vi "Destroy.vi"(8 "error in (no error)":errorcluster, 11 "StartupSplash in":refnum<class "StartupSplash.lvclass">) -> (0 "error out":errorcluster)   [LabVIEW 2025, in "StartupSplash.lvclass"]
uses:
  StartupSplash.lvclass
  StartupSplash.lvclass/StartupSplash.ctl
  zeromq/Send_string.vi
  zeromq/Socket.lvclass
  zeromq/Context.lvclass
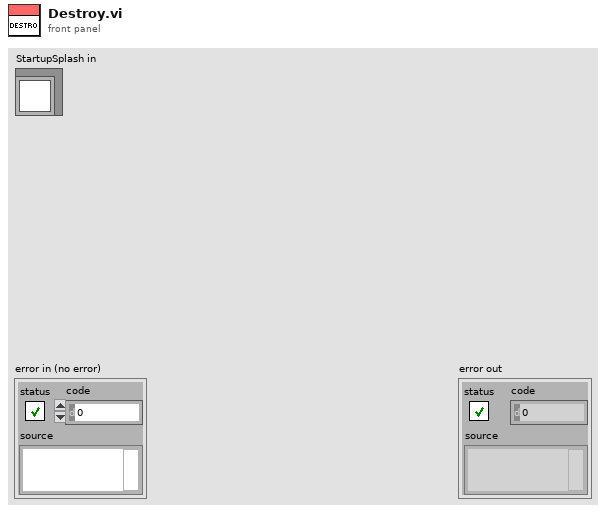
[diagram p1: front panel]
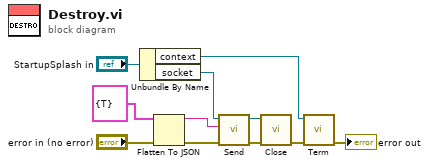
[diagram p0: block diagram]
diagram:
  n1 = Unbundle By Name("StartupSplash in") -> ("context"=w10:refnum<class "Context.lvclass">, "socket"=w6:refnum<class "Socket.lvclass">)
  n2 = Flatten To JSON(anything=cluster{"done":bool} {"done"=TRUE}, error in (no error)="error in (no error)") -> (JSON string=w4:string, 11:w3:errorcluster)  [unwired: 1 in]
  n3 = call-poly "Send.vi"("error in"=w3, "data"=w4, "socket in"=w6) -> ("error out"=w1:errorcluster, "socket out"=w5:refnum<class "Socket.lvclass">)  [unwired: 7 in]
  n4 = call "Close.vi"("error in"=w1, "socket"=w5) -> ("error out"=w9:errorcluster)  [unwired: 9 in]
  n5 = call "Term.vi"("error in"=w9, "context in"=w10) -> ("error out"=→"error out":errorcluster)  [unwired: 9 in]
